vi "4. SJCubeRunExp.vi"() -> ()   [LabVIEW 2019, in "SJCube_KNRm.lvlib"]
uses:
  SJCube_KNRm.lvlib
  PendulumState.ctl
  KNRm_ReMi_OS5.lvlibp/KNRm_ReMi_Toolkit/IO/LowLevel/IO_Channel_DIO.ctl
  <vilib>/Platform/TimedLoop/XDataNode/timing_clust.ctl
  <vilib>/Platform/TimedLoop/XDataNode/nitl_modes.ctl
  <vilib>/Platform/TimedLoop/XDataNode/wakeup.ctl
  <vilib>/myRIO/Common/Instrument Driver Framework/myRIO v1.0/UART/vis/myRIO v1.0 Close UART.vi
  <vilib>/addons/control/pid/pid.llb/PID (DBL).vi
  <vilib>/myRIO/Common/Instrument Driver Framework/Utilities/vis/FPGA Ref Manager.vi
  <vilib>/myRIO/Common/Instrument Driver Framework/myRIO v1.0/myRIO v1.0 Reset FPGA.vi
  <vilib>/myRIO/Common/Instrument Driver Framework/myRIO v1.0/IRQ/vis/myRIO v1.0 IRQ Info FGV.vi
  <vilib>/myRIO/Common/Instrument Driver Framework/myRIO v1.0/IRQ/vis/myRIO v1.0 Timer IRQ Info FGV.vi
  <vilib>/myRIO/Common/Instrument Driver Framework/myRIO v1.0/IRQ/vis/myRIO v1.0 ISR Agent.vi
  <vilib>/myRIO/Instrument Drivers/Utilities/vis/Reset Index.vi
  <vilib>/myRIO/Common/Instrument Driver Framework/myRIO v1.0/Resource Manager/vis/myRIO v1.0 Block Write Resource Manager.vi
  <vilib>/Platform/TimedLoop/XDataNode/XDataNode.xnode
  <vilib>/Platform/TimedLoop/XDataNode/XDNodeRunTimeDep.lvlib
  <vilib>/myRIO/Instrument Drivers/Utilities/Utilities.lvlib
  <vilib>/ptbypt/NI_PtbyPt.lvlib
  <vilib>/addons/control/pid/NI_PID_pid.lvlib
  KNRm_ReMi_OS5.lvlibp
panel:
  in  "Stop Button 2":bool
  in  "motorPID":T1={"proportional gain (Kc)"=2.0, "integral time (Ti, min)"=0.0, "derivative time (Td, min)"=0.0005}
  in  "PosPID":T1={"proportional gain (Kc)"=-0.05999999999999999, "integral time (Ti, min)"=0.05, "derivative time (Td, min)"=0.019999999999999997}
  in  "BalancePID":T1={"proportional gain (Kc)"=0.07999999999999999, "integral time (Ti, min)"=0.0, "derivative time (Td, min)"=0.0006}
  out "nowState":T2
  in  "NextState":T2
  in  "manual State":bool
  out "Waveform Chart":T3(graph)
  in  "Setpoint(deg)":dbl(knob) scale=80.0..-80.0
  out "error out":errorcluster
  out "Position(deg)":dbl(knob) scale=80.0..-80.0
  in  "Reset":bool
  in  "Stop Button":bool
  out "MotorResetPOS":dbl[](array[numeric])
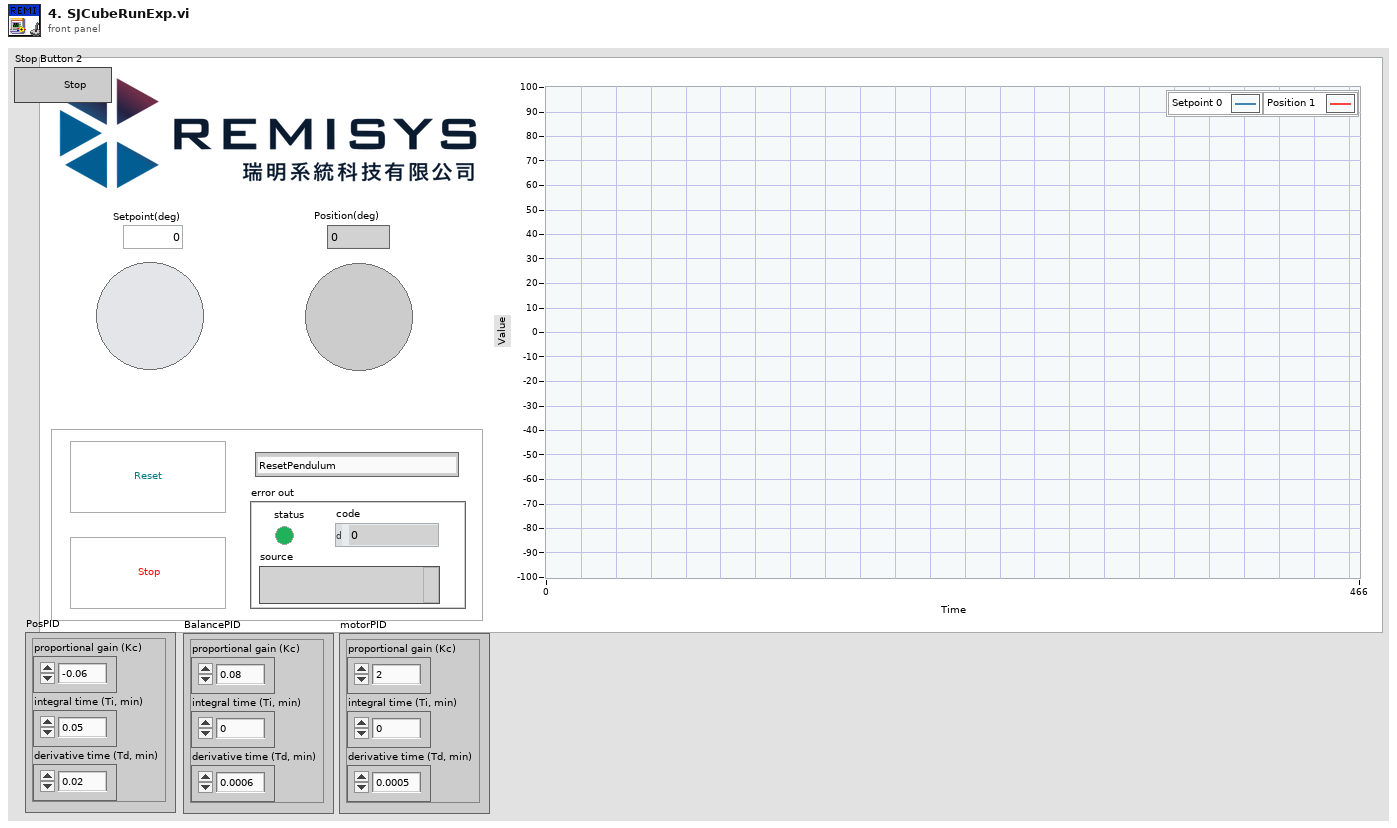
[diagram p1: front panel]
types:
  T1 = cluster{"proportional gain (Kc)":dbl, "integral time (Ti, min)":dbl, "derivative time (Td, min)":dbl}
  T2 = typedef "SJCube_KNRm.lvlib/PendulumState.ctl" = enum16{"ResetPendulum", "PendulumFindHome", "PendulumToHome", "SwingUp", "Balancing", "ExitExp."}
  T3 = cluster{"Setpoint(deg)":dbl, "PresentPOS(deg)":dbl}
  T4 = typedef "KNRm_ReMi_OS5.lvlibp/IO_Channel_DIO.ctl" = enum16{"B/DIO1 (M1)", "A/DIO8 (M2)", "B/DIO7 (M3)", "A/DIO3 (M4)", "A/DIO14 (RC1_0)", "A/DIO15 (RC1_1)"}
  T5 = typedef "XDNodeRunTimeDep.lvlib/timing_clust.ctl" = cluster{"Expected End [f-1]":u64, "Actual End [f-1]":u64, "Finished Late? [f-1]":bool, "Expected End [i-1]":u64, "Actual End [i-1]":u64, "Finished Late? [i-1]":bool, "Expected Start [i]":u64, "Actual Start [i]":u64, "Expected Start [f]":u64, "Actual Start [f]":u64, "Source Name":string, "Structure Name":string, "Period":i64, "Deadline":i64, "Offset":i64, "Start":i64, "Priority":i32, "Timeout":i32, "Mode":T6, "Wakeup Reason":T7, "Error":errorcluster, "Source Type":string, "Secondary Source Type":string, "Global End Time":u64, "Global Start Time":u64, "Frame Duration":u64, "Iteration Duration":u64, "Assigned CPU":i32, "I/O Scan Engine Mode":u32}
  T6 = typedef "XDNodeRunTimeDep.lvlib/nitl_modes.ctl" = enum32{"No Change", "Process missed periods, maintain original phase", "Discard missed periods, maintain original phase", "Process missed periods, ignore original phase", "Discard missed periods, ignore original phase"}
  T7 = typedef "XDNodeRunTimeDep.lvlib/wakeup.ctl" = enum32{"Normal", "Aborted", "Asynchronous wakeup", "Timing source error", "Timed loop error", "Timeout"}
  T8 = cluster{"Setpoint(deg)":dbl, "MotorEncoder (deg)":dbl}
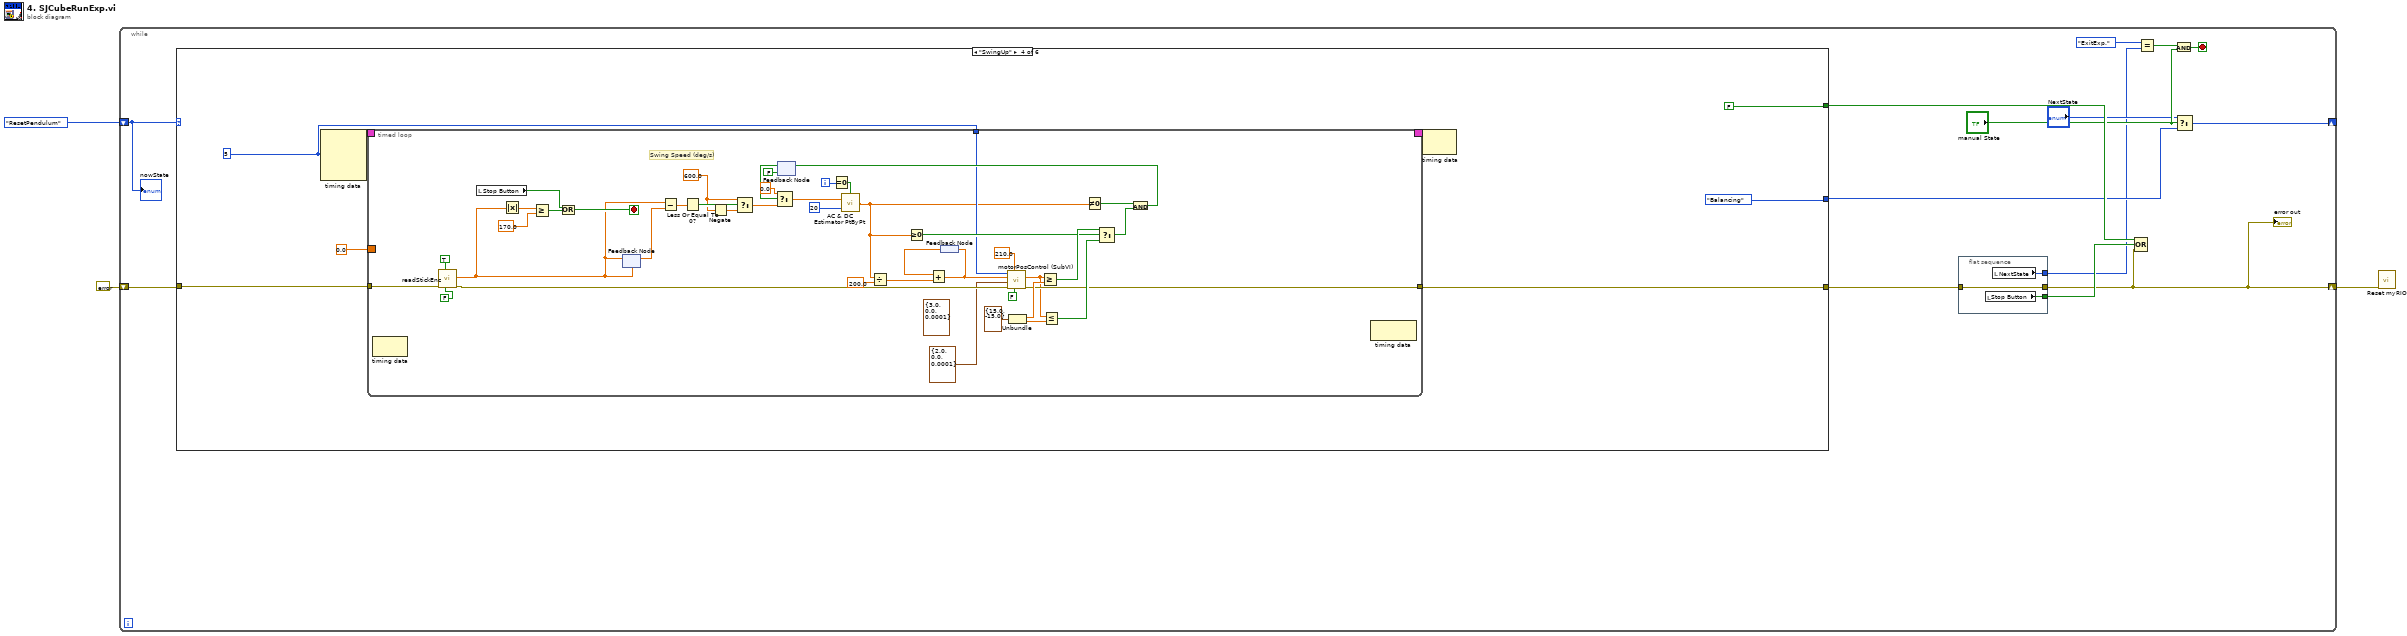
[diagram p0: block diagram]
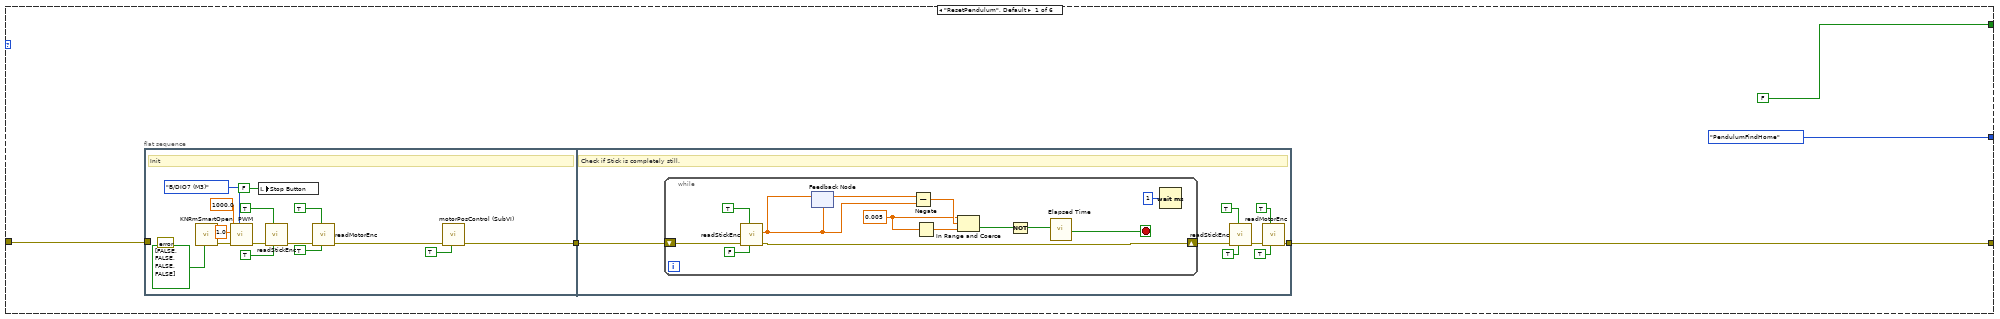
[diagram p2: hidden frame]
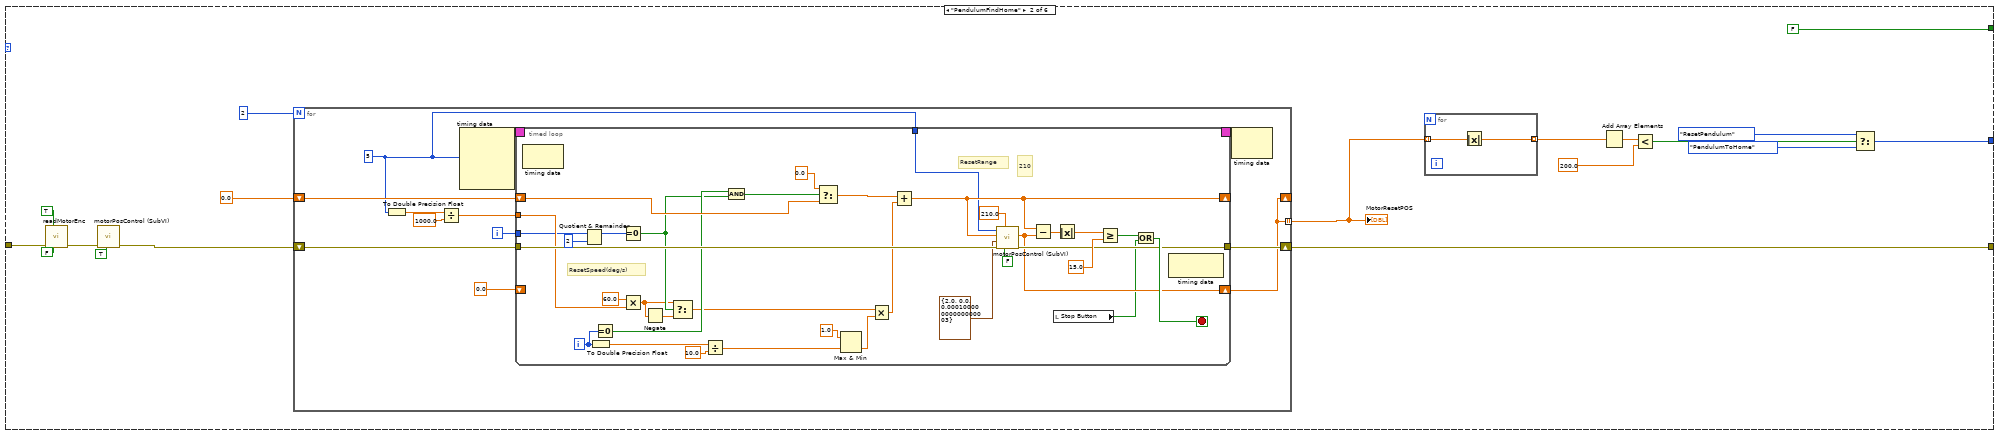
[diagram p3: hidden frame]
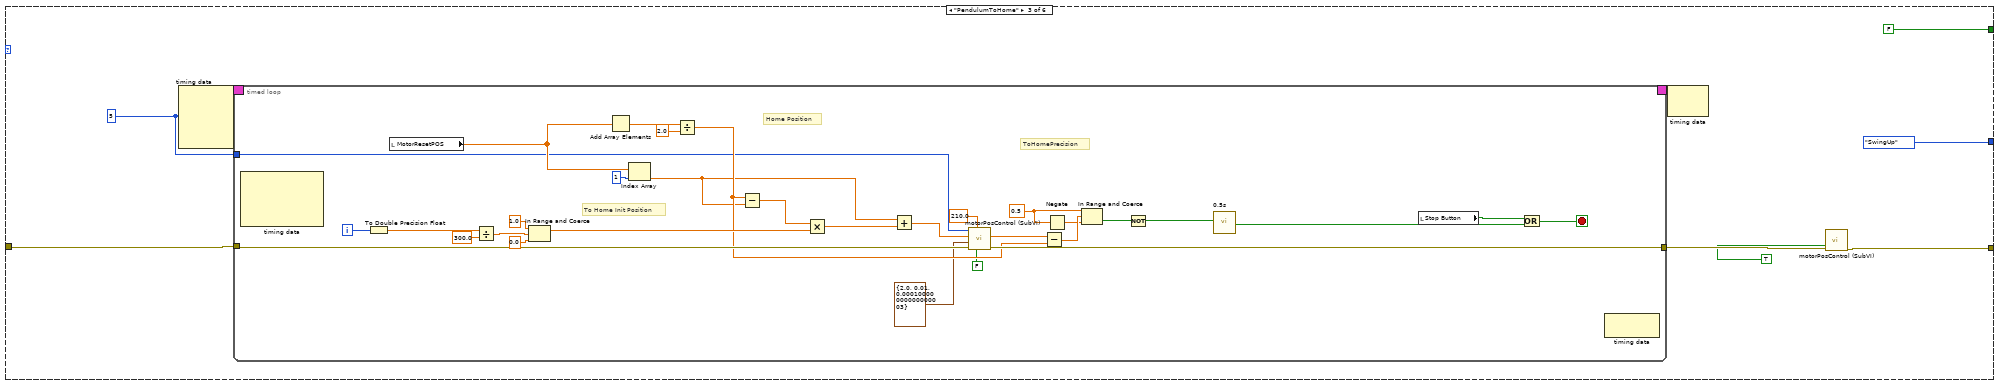
[diagram p4: hidden frame]
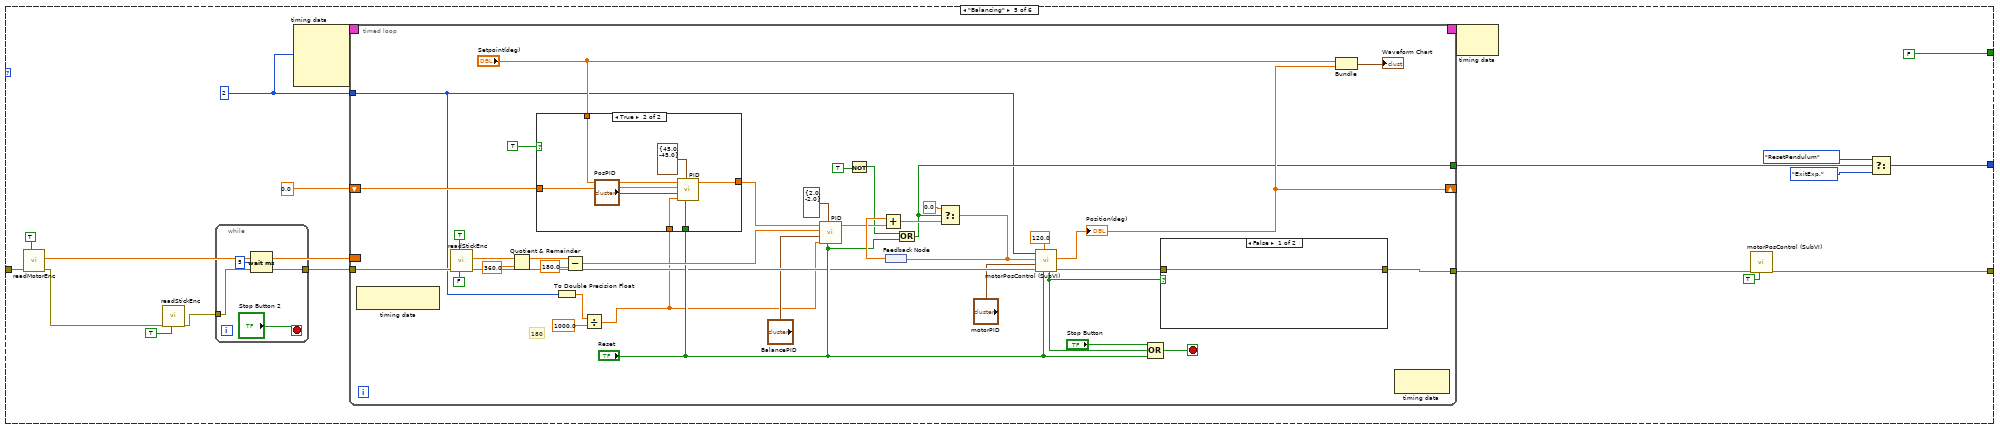
[diagram p5: hidden frame]
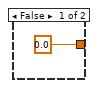
[diagram p6: hidden frame]
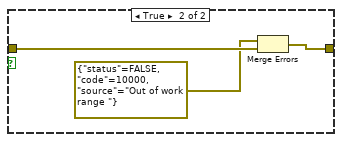
[diagram p7: hidden frame]
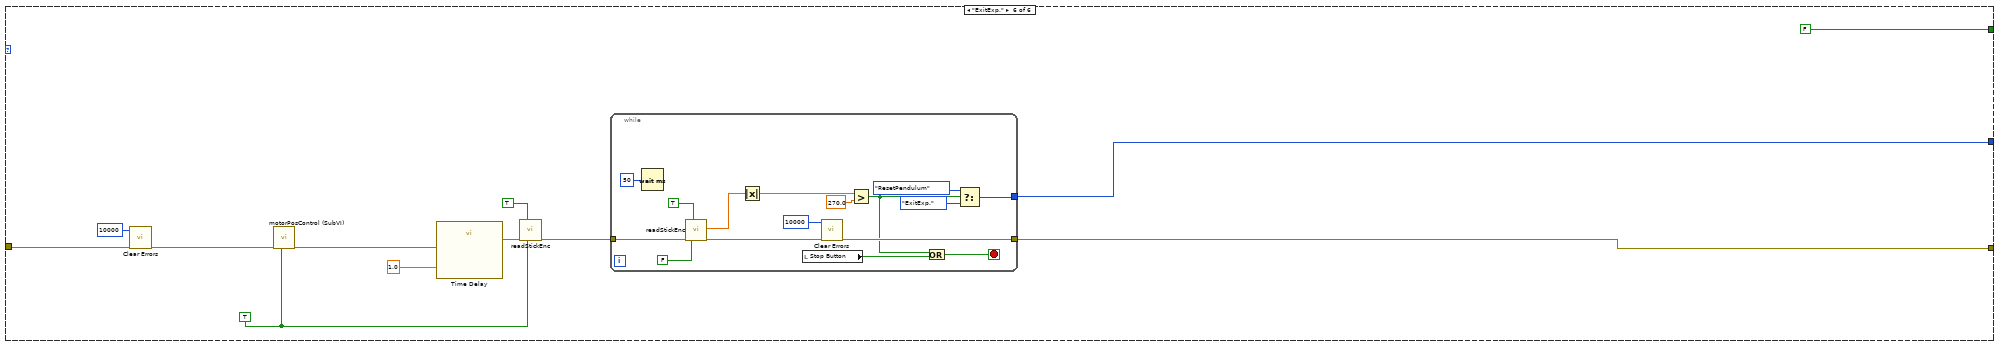
[diagram p8: hidden frame]
diagram:
  n1 = while {
    shift-right: [w11] -> _
    shift-left: PendulumState."ResetPendulum" ("Start State") -> [w13]
    shift-right: [w4] -> w1
    shift-left: errorcluster {"status"=FALSE, "code"=0, "source"=""} ("error in (no error)") -> [w17]
    stop <- w7 stop-if-true
    n2 = case shown="\"SwingUp\"" w13 {
      tunnel: w17 -> [w23 w76 w140 w184 w243 w323]
      tunnel: [w24 w79 w137 w183 w255 w321] -> w16
      tunnel: [PendulumState."PendulumFindHome" w62 PendulumState."SwingUp" PendulumState."Balancing" w252 w325] -> w12
      tunnel: [FALSE FALSE FALSE FALSE FALSE FALSE] -> w14
      frame "ResetPendulum", Default {
        n3 = flat-sequence {
          tunnel: w23 -> [_]
          tunnel: [w33] -> w21
          tunnel: [w44] -> w24
          tunnel: w21 -> [w41]
          frame #0 {
            (unwired) errorcluster {"status"=FALSE, "code"=0, "source"=""} ("error in (no error)")
            # "Init"
            n4 = call "KNRmSmartOpen.vi"("SpeedMode"=bool[] [FALSE, FALSE, FALSE, FALSE]) -> ("error out"=w30:errorcluster)  [unwired: 8 in, 2 out]
            n5 = call "PWM.vi"("IO_Chanel"=IO_Channel_DIO."B/DIO7 (M3)", "error in"=w30, "DutyCycle"=1.0, "Frequency(Hz)"=1000.0) -> ("error out"=w29:errorcluster)  [unwired: 7 in]
            n6 = local write "Stop Button"(FALSE ("Stop Button")) -> ()
            n7 = call "readStickEnc.vi"("Reset Counter"=TRUE, "Reverse ENC?"=TRUE, "error in (no error)"=w29) -> ("error out"=w37:errorcluster)  [unwired: 7 in, 1 out]
            n8 = call "readMotorEnc.vi"("Reset Counter"=TRUE, "Reverse ENC?"=TRUE, "error in (no error)"=w37) -> ("error out"=w34:errorcluster)  [unwired: 7 in, 1 out]
            n9 = call "motorPosControl (SubVI).vi"("Reset"=TRUE, "error in (no error)"=w34) -> ("error out"=w33:errorcluster)  [unwired: 6 in, 3 out]
          }
          frame #1 {
            # "Check if Stick is completely still."
            n10 = while {
              shift-right: [w61] -> w48
              shift-left: w41 -> [w60]
              stop <- w51 stop-if-true
              w57 = 0.005 ("upper limit")
              n11 = call "readStickEnc.vi"("Reset Counter"=FALSE, "Reverse ENC?"=TRUE, "error in (no error)"=w60) -> ("error out"=w61:errorcluster, "StickEncoder (deg)"=w55:dbl)  [unwired: 7 in]
              n12 = feedback-in #1(w55) -> ()
              n13 = feedback #1(w55) -> (w59:dbl)
              n14 = Subtract(x=w59, y=w55) -> (x-y=w58:dbl)
              n15 = Negate(x=w57) -> (-x=w56:dbl)
              n16 = In Range and Coerce(upper limit=w57, x=w58, lower limit=w56) -> (In Range?=w53:bool)  [unwired: 1 out]
              n17 = Not(x=w53) -> (.not. x?=w52:bool)
              n18 = call "Elapsed Time"("Reset"=w52) -> ("Time has Elapsed"=w51:bool)  [unwired: 11 in, 7 out]
              n19 = Wait (ms)(milliseconds to wait=u32 1) -> ()  [unwired: 1 out]
            }
            n20 = call "readStickEnc.vi"("Reset Counter"=TRUE, "Reverse ENC?"=TRUE, "error in (no error)"=w48) -> ("error out"=w45:errorcluster)  [unwired: 7 in, 1 out]
            n21 = call "readMotorEnc.vi"("Reset Counter"=TRUE, "Reverse ENC?"=TRUE, "error in (no error)"=w45) -> ("error out"=w44:errorcluster)  [unwired: 7 in, 1 out]
          }
        }
      }
      frame "PendulumFindHome" {
        n22 = call "readMotorEnc.vi"("Reset Counter"=FALSE, "Reverse ENC?"=TRUE ("Reset Button"), "error in (no error)"=w76) -> ("error out"=w77:errorcluster)  [unwired: 7 in, 1 out]
        n23 = call "motorPosControl (SubVI).vi"("Reset"=TRUE, "error in (no error)"=w77) -> ("error out"=w71:errorcluster)  [unwired: 6 in, 3 out]
        n24 = for {
          N: 2 -> [_]
          shift-right: [w91] -> w79
          shift-left: w71 -> [w90]
          shift-right: [w84] -> _
          shift-left: 0.0 ("PresentPOS(deg)") -> [w88]
          tunnel: [w84] -> w69 mode=indexing
          i -> [w89]
          w82 = i64 5 ("Period")
          n25 = To Double Precision Float(number=w82) -> (double precision float=w87:dbl)
          n26 = Divide(x=w87, y=1000.0) -> (x/y=w85:dbl)
          n27 = node-c288(w82) -> (w93:T5)  [unwired: 3 in]
          n28 = timed-loop {
            timing: w93 -> [_]
            timing-out: [_] -> w92
            tunnel: w90 -> [w123]
            tunnel: [w122] -> w91
            tunnel: w89 -> [w107]
            shift-right: [w118] -> _
            shift-left: w88 -> [w106]
            tunnel: w85 -> [w114]
            shift-right: [w113] -> w84
            shift-left: 0.0 ("MotorEncoder (deg)") -> [_]
            tunnel: w82 -> [w95]
            i -> [w102]
            stop <- w127 stop-if-true
            # "210"
            # "ResetRange"
            # "ResetSpeed(deg/s)"
            n29 = node-c288() -> ()  [unwired: 1 in, 1 out]
            n30 = Quotient & Remainder(x=w107, y=2) -> (x-y*floor(x/y)=w103:i32)  [unwired: 1 out]
            n31 = To Double Precision Float(number=w102) -> (double precision float=w119:dbl)
            n32 = Equal To 0?(x=w102) -> (x = 0?=w100:bool)
            n33 = Equal To 0?(x=w103) -> (x = 0?=w99:bool)
            n34 = Multiply(x=60.0 ("y"), y=w114) -> (x*y=w98:dbl)
            n35 = Negate(x=w98) -> (-x=w97:dbl)
            n36 = Select(t=w98, s=w99, f=w97) -> (s? t:f=w96:dbl)
            n37 = Divide(x=w119, y=10.0) -> (x/y=w117:dbl)
            n38 = And(x=w100, y=w99) -> (x .and. y?=w101:bool)
            n39 = Select(t=0.0, s=w101, f=w106) -> (s? t:f=w104:dbl)
            n40 = Max & Min(x=1.0 ("upper limit"), y=w117) -> (min(x,y)=w112:dbl)  [unwired: 1 out]
            n41 = Multiply(x=w96, y=w112) -> (x*y=w109:dbl)
            n42 = Add(x=w104, y=w109) -> (x+y=w118:dbl)
            n43 = call "motorPosControl (SubVI).vi"("Reset"=FALSE, "+/- Range"=210.0 ("WorkRange"), "error in (no error)"=w123, "PID gains"=T1 {"proportional gain (Kc)"=2.0, "integral time (Ti, min)"=0.0, "derivative time (Td, min)"=0.00010000000000000003}, "Position (deg)"=w118, "dt"=w95) -> ("error out"=w122:errorcluster, "MotorEncoder (deg)"=w113:dbl)  [unwired: 2 in, 2 out]
            n44 = Subtract(x=w118, y=w113) -> (x-y=w125:dbl)
            n45 = local read "Stop Button"() -> (w110:bool)
            n46 = Absolute Value(x=w125) -> (abs(x)=w124:dbl)
            n47 = Greater Or Equal?(x=w124, y=15.0) -> (x >= y?=w111:bool)
            n48 = Or(x=w111, y=w110) -> (x .or. y?=w127:bool)
            n49 = node-c288() -> ()  [unwired: 1 in, 1 out]
          }
          n50 = node-c288(w92) -> ()  [unwired: 1 out]
        }
        "MotorResetPOS" <- w69
        n51 = for {
          tunnel: w69 -> [w81] mode=indexing
          tunnel: [w80] -> w68 mode=indexing
          n52 = Absolute Value(x=w81) -> (abs(x)=w80:dbl)
        }
        n53 = Add Array Elements(numeric array=w68) -> (sum=w67:dbl)
        n54 = Less?(x=w67, y=200.0) -> (x < y?=w65:bool)
        n55 = Select(t=PendulumState."ResetPendulum", s=w65, f=PendulumState."PendulumToHome") -> (s? t:f=w62:T2)
      }
      frame "PendulumToHome" {
        w135 = i64 5 ("Period")
        n56 = node-c288(w135) -> (w142:T5)  [unwired: 3 in]
        n57 = timed-loop {
          timing: w142 -> [_]
          timing-out: [_] -> w141
          tunnel: w140 -> [w174]
          tunnel: [w169] -> w139
          tunnel: w135 -> [w144]
          i -> [w168]
          stop <- w154 stop-if-true
          w171 = 0.5
          # "To Home Init Position"
          # "Home Position"
          # "ToHomePrecision"
          n58 = node-c288() -> ()  [unwired: 1 in, 4 out]
          n59 = To Double Precision Float(number=w168) -> (double precision float=w151:dbl)
          n60 = local read "MotorResetPOS"() -> (w163:dbl[])
          n61 = Divide(x=w151, y=300.0) -> (x/y=w166:dbl)
          n62 = In Range and Coerce(upper limit=1.0, x=w166, lower limit=0.0) -> (coerced(x)=w161:dbl)  [unwired: 1 out]
          n63 = Add Array Elements(numeric array=w163) -> (sum=w162:dbl)
          n64 = Index Array(array=w163, index=1) -> (element=w157:dbl)
          n65 = Divide(x=w162, y=2.0) -> (x/y=w159:dbl)
          n66 = Subtract(x=w159, y=w157) -> (x-y=w158:dbl)
          n67 = Multiply(x=w158, y=w161) -> (x*y=w160:dbl)
          n68 = Add(x=w157, y=w160) -> (x+y=w156:dbl)
          n69 = call "motorPosControl (SubVI).vi"("Reset"=FALSE, "+/- Range"=210.0 ("WorkRange"), "error in (no error)"=w174, "PID gains"=T1 {"proportional gain (Kc)"=2.0, "integral time (Ti, min)"=0.01, "derivative time (Td, min)"=0.00010000000000000003}, "Position (deg)"=w156, "dt"=w144) -> ("error out"=w169:errorcluster, "MotorEncoder (deg)"=w173:dbl)  [unwired: 2 in, 2 out]
          n70 = Subtract(x=w173, y=w159) -> (x-y=w172:dbl)
          n71 = Negate(x=w171) -> (-x=w170:dbl)
          n72 = In Range and Coerce(upper limit=w171, x=w172, lower limit=w170) -> (In Range?=w149:bool)  [unwired: 1 out]
          n73 = Not(x=w149) -> (.not. x?=w148:bool)
          n74 = call "0.5s"("Reset"=w148) -> ("Time has Elapsed"=w146:bool)  [unwired: 11 in, 7 out]
          n75 = local read "Stop Button"() -> (w145:bool)
          n76 = Or(x=w145, y=w146) -> (x .or. y?=w154:bool)
          n77 = node-c288() -> ()  [unwired: 1 in, 1 out]
        }
        n78 = node-c288(w141) -> ()  [unwired: 1 out]
        n79 = call "motorPosControl (SubVI).vi"("Reset"=TRUE ("Reset Button"), "error in (no error)"=w139) -> ("error out"=w137:errorcluster)  [unwired: 6 in, 3 out]
      }
      frame "SwingUp" {
        w181 = i64 5 ("Period")
        n80 = node-c288(w181) -> (w186:T5)  [unwired: 3 in]
        n81 = timed-loop {
          timing: w186 -> [_]
          timing-out: [_] -> w185
          tunnel: w184 -> [w210]
          tunnel: [w209] -> w183
          border: 0.0 -> [_]
          tunnel: w181 -> [w192]
          i -> [w231]
          stop <- w227 stop-if-true
          (unwired) T1 {"proportional gain (Kc)"=3.0, "integral time (Ti, min)"=0.0, "derivative time (Td, min)"=0.0001} ("PID gains")
          w223 = 600.0 ("MaxSpeed(deg/s)")
          # "Swing Speed (deg/s)"
          n82 = node-c288() -> ()  [unwired: 1 in, 1 out]
          n83 = call "readStickEnc.vi"("Reset Counter"=FALSE, "Reverse ENC?"=TRUE, "error in (no error)"=w210) -> ("error out"=w207:errorcluster, "StickEncoder (deg)"=w201:dbl)  [unwired: 7 in]
          n84 = local read "Stop Button"() -> (w205:bool)
          n85 = Absolute Value(x=w201) -> (abs(x)=w229:dbl)
          n86 = Greater Or Equal?(x=w229, y=170.0) -> (x >= y?=w206:bool)
          n87 = Or(x=w205, y=w206) -> (x .or. y?=w227:bool)
          n88 = feedback-in #2(w201) -> ()
          n89 = feedback #2(w201) -> (w230:dbl)
          n90 = Subtract(x=w201, y=w230) -> (x-y=w226:dbl)
          n91 = Less Or Equal To 0?(x=w226) -> (x <= 0?=w225:bool)
          n92 = Negate(x=w223) -> (-x=w224:dbl)
          n93 = Select(t=w223, s=w225, f=w224) -> (s? t:f=w191:dbl)
          n94 = feedback #3(FALSE) -> (w220:bool)
          n95 = Select(t=0.0, s=w220, f=w191) -> (s? t:f=w200:dbl)
          n96 = Equal To 0?(x=w231) -> (x = 0?=w195:bool)
          n97 = call <vilib>:"AC & DC Estimator PtByPt.vi"("signal"=w200, "sample length"=20, "initialize"=w195) -> ("DC estimate (V)"=w190:dbl)  [unwired: 2 out]
          n98 = Divide(x=w190, y=200.0 ("x")) -> (x/y=w199:dbl)
          n99 = Greater Or Equal To 0?(x=w190) -> (x >= 0?=w204:bool)
          n100 = feedback #4() -> (w222:dbl)
          n101 = Add(x=w222, y=w199) -> (x+y=w198:dbl)
          n102 = feedback-in #4(w198) -> ()
          n103 = call "motorPosControl (SubVI).vi"("Reset"=FALSE, "+/- Range"=210.0 ("WorkRange"), "error in (no error)"=w207, "PID gains"=T1 {"proportional gain (Kc)"=2.0, "integral time (Ti, min)"=0.0, "derivative time (Td, min)"=0.0001}, "Position (deg)"=w198, "dt"=w192) -> ("error out"=w209:errorcluster, "MotorEncoder (deg)"=w202:dbl)  [unwired: 2 in, 2 out]
          n104 = Unbundle(cluster{"UpLimit":dbl, "DownLimit":dbl} {"UpLimit"=15.0, "DownLimit"=-15.0} ("RunUpLimuit")) -> ("UpLimit"=w217:dbl, "DownLimit"=w216:dbl)
          n105 = Greater Or Equal?(x=w202, y=w217) -> (x >= y?=w215:bool)
          n106 = Less Or Equal?(x=w202, y=w216) -> (x <= y?=w214:bool)
          n107 = Not Equal To 0?(x=w190) -> (x != 0?=w213:bool)
          n108 = Select(t=w215, s=w204, f=w214) -> (s? t:f=w212:bool)
          n109 = And(x=w213, y=w212) -> (x .and. y?=w203:bool)
          n110 = feedback-in #3(w203) -> ()
          n111 = node-c288() -> ()  [unwired: 1 in, 1 out]
        }
        n112 = node-c288(w185) -> ()  [unwired: 1 out]
      }
      frame "Balancing" {
        w245 = i64 2 ("Period")
        n113 = call "readMotorEnc.vi"("Reverse ENC?"=TRUE, "error in (no error)"=w243) -> ("error out"=w241:errorcluster, "MotorEncoder (deg)"=w242:dbl)  [unwired: 8 in]
        n114 = call "readStickEnc.vi"("Reset Counter"=TRUE, "error in (no error)"=w241) -> ("error out"=w239:errorcluster)  [unwired: 8 in, 1 out]
        n115 = while {
          tunnel: w239 -> [w259]
          tunnel: [w259] -> w238
          stop <- "Stop Button 2" stop-if-true
          n116 = Wait (ms)(milliseconds to wait=u32 5) -> ()  [unwired: 1 out]
        }
        n117 = node-c288(w245) -> (w250:T5)  [unwired: 3 in]
        n118 = timed-loop "Timed Loop" {
          timing: w250 -> [_]
          timing-out: [_] -> w249
          border: w242 -> [_]
          shift-right: [w268] -> _
          shift-left: 0.0 -> [w269]
          tunnel: w238 -> [w276]
          tunnel: [w266] -> w247
          tunnel: [w274] -> w246
          tunnel: w245 -> [w260]
          stop <- w286 stop-if-true
          # "180"
          n119 = node-c288() -> ()  [unwired: 1 in, 1 out]
          n120 = call "readStickEnc.vi"("Reset Counter"=FALSE, "Reverse ENC?"=TRUE, "error in (no error)"=w276) -> ("error out"=w278:errorcluster, "StickEncoder (deg)"=w279:dbl)  [unwired: 7 in]
          n121 = Quotient & Remainder(x=w279, y=360.0) -> (x-y*floor(x/y)=w287:dbl)  [unwired: 1 out]
          n122 = To Double Precision Float(number=w260) -> (double precision float=w261:dbl)
          n123 = Subtract(x=w287, y=180.0) -> (x-y=w292:dbl)
          n124 = Divide(x=w261, y=1000.0) -> (x/y=w262:dbl)
          n125 = case shown="True" TRUE ("StickPosControl") {
            tunnel: w262 -> [_ w304]
            tunnel: [0.0 ("output") w302] -> w289
            tunnel: w269 -> [_ w301]
            tunnel: "Reset" -> [_ w300]
            tunnel: "Setpoint(deg)" -> [_ w298]
            frame False {
            }
            frame True {
              n126 = call-poly <vilib>:"PID.vi"("reinitialize? (F)"=w300, "output range"=cluster{"output high":dbl, "output low":dbl} {"output high"=45.0, "output low"=-45.0}, "dt (s)"=w304, "PID gains"="PosPID", "process variable"=w301, "setpoint"=w298) -> ("output"=w302:dbl)  [unwired: 4 in, 1 out]
            }
          }
          n127 = call-poly <vilib>:"PID.vi"("reinitialize? (F)"="Reset", "output range"=cluster{"output high":dbl, "output low":dbl} {"output high"=2.0, "output low"=-2.0}, "dt (s)"=w262, "PID gains"="BalancePID", "process variable"=w292, "setpoint"=w289) -> ("output"=w290:dbl)  [unwired: 4 in, 1 out]
          n128 = Not(x=TRUE ("BalanceControl")) -> (.not. x?=w264:bool)
          n129 = feedback #5() -> (w295:dbl)
          n130 = Add(x=w295, y=w290) -> (x+y=w294:dbl)
          n131 = Or(x=w264, y="Reset") -> (x .or. y?=w266:bool)
          n132 = Select(t=0.0, s=w266, f=w294) -> (s? t:f=w281:dbl)
          n133 = feedback-in #5(w281) -> ()
          n134 = call "motorPosControl (SubVI).vi"("Reset"="Reset", "+/- Range"=120.0 ("WorkRange"), "error in (no error)"=w278, "PID gains"="motorPID", "Position (deg)"=w281, "dt"=w260) -> ("error out"=w283:errorcluster, "MotorEncoder (deg)"=w268:dbl, "out of range!"=w284:bool)  [unwired: 2 in, 1 out]
          "Position(deg)" <- w268
          n135 = Compound Arithmetic op=OR("Stop Button", w284, "Reset") -> (w286:bool)
          n136 = case shown="False" w284 {
            tunnel: w283 -> [w305 w308]
            tunnel: [w305 w307] -> w274
            frame False {
            }
            frame True {
              n137 = Merge Errors(errorcluster {"status"=FALSE, "code"=10000, "source"="Out of work range "} ("error in (no error)"), w308) -> (w307:errorcluster)
            }
          }
          n138 = Bundle("Setpoint(deg)"="Setpoint(deg)", "MotorEncoder (deg)"=w268) -> (→"Waveform Chart":T8)  [unwired: 1 in]
          n139 = node-c288() -> ()  [unwired: 1 in, 1 out]
        }
        n140 = node-c288(w249) -> ()  [unwired: 1 out]
        n141 = call "motorPosControl (SubVI).vi"("Reset"=TRUE ("Reset Button"), "error in (no error)"=w246) -> ("error out"=w255:errorcluster)  [unwired: 6 in, 3 out]
        n142 = Select(t=PendulumState."ResetPendulum", s=w247, f=PendulumState."ExitExp.") -> (s? t:f=w252:T2)
      }
      frame "ExitExp." {
        w318 = TRUE ("Reset Counter")
        n143 = call <vilib>:"Clear Errors.vi"("error in (no error)"=w323, "specific error code to clear (0: all)"=10000) -> ("error out"=w320:errorcluster)  [unwired: 4 in, 1 out]
        n144 = call "motorPosControl (SubVI).vi"("Reset"=w318, "error in (no error)"=w320) -> ("error out"=w319:errorcluster)  [unwired: 6 in, 3 out]
        n145 = call "Time Delay"("error in (no error)"=w319, "Delay Time (s)"=1.0) -> ("error out"=w317:errorcluster)  [unwired: 9 in]
        n146 = call "readStickEnc.vi"("Reset Counter"=w318, "Reverse ENC?"=TRUE, "error in (no error)"=w317) -> ("error out"=w316:errorcluster)  [unwired: 7 in, 1 out]
        n147 = while {
          tunnel: w316 -> [w342]
          tunnel: [w336] -> w325
          tunnel: [w332] -> w321
          stop <- w329 stop-if-true
          n148 = Wait (ms)(milliseconds to wait=u32 50) -> ()  [unwired: 1 out]
          n149 = call "readStickEnc.vi"("Reset Counter"=FALSE, "Reverse ENC?"=TRUE, "error in (no error)"=w342) -> ("error out"=w333:errorcluster, "StickEncoder (deg)"=w339:dbl)  [unwired: 7 in]
          n150 = Absolute Value(x=w339) -> (abs(x)=w331:dbl)
          n151 = local read "Stop Button"() -> (w328:bool)
          n152 = call <vilib>:"Clear Errors.vi"("error in (no error)"=w333, "specific error code to clear (0: all)"=10000) -> ("error out"=w332:errorcluster)  [unwired: 4 in, 1 out]
          n153 = Greater?(x=w331, y=270.0) -> (0:w327:bool)
          n154 = Or(x=w327, y=w328) -> (x .or. y?=w329:bool)
          n155 = Select(t=PendulumState."ResetPendulum", s=w327, f=PendulumState."ExitExp.") -> (s? t:f=w336:T2)
        }
      }
    }
    n156 = flat-sequence {
      tunnel: w16 -> [w19]
      tunnel: [w20] -> w15
      tunnel: [w19] -> w4
      tunnel: [w18] -> w5
      frame #0 {
        n157 = local read "Stop Button"() -> (w20:bool)
        n158 = local read "NextState"() -> (w18:T2)
      }
    }
    n159 = Compound Arithmetic op=OR(w14, w15, w4) -> ()  [unwired: 1 out]
    n160 = Equal?(x=PendulumState."ExitExp." ("y"), y=w5) -> (x = y?=w8:bool)
    n161 = And(x=w8, y="manual State") -> (x .and. y?=w7:bool)
    n162 = Select(t="NextState", s="manual State", f=w12) -> (s? t:f=w11:T2)
    "error out" <- w4
    "nowState" <- w13
  }
  n163 = call <vilib>:"Reset myRIO.vi"("error in (no error)"=w1) -> ()  [unwired: 10 in, 1 out]
